vi "dfd_Draw Polynomial Matrix Element.vi"(4 "format control":T1={"variable"="z", "rendering options"={"coefficients ascending order"=FALSE, "render ascending order"=TRUE, "negative exponent"=TRUE}}, 5 "fonts input":T5(array[cluster]), 6 "alignment(left, top)":T4, 7 "format string":string="%#.4g", 9 "origin":cluster{"x":i16, "y":i16}, 10 "coefficients":dbl[](array[numeric])=[1.0, 2.0, 1.0, 0.0, 2.0] format="%.2f", 11 "picture in":picture) -> (1 "location":T3, 3 "picture out":picture)   [LabVIEW 2017, in "NI_DigFilter_Process.lvlib"]
uses:
  <vilib>/addons/Digital Filter Design/NI_DigFilter_Process.lvlib
  <vilib>/Analysis/polynomials.llb/Remove Zero Coefficients (DBL).vi
  <vilib>/Analysis/NI_AALPro.lvlib
panel:
  in  "desired font(user-specified font)":T2(ring)
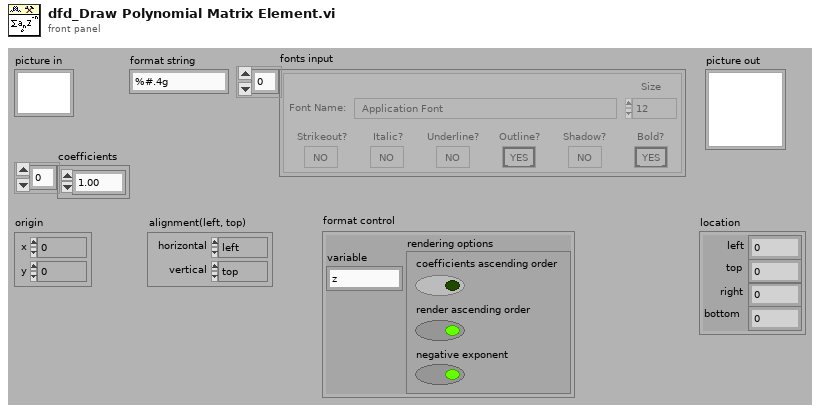
[diagram p1: front panel]
types:
  T1 = cluster{"variable":string, "rendering options":cluster{"coefficients ascending order":bool, "render ascending order":bool, "negative exponent":bool}}
  T2 = enum16{"User-specified Font", "Application Font", "System Font", "Dialog Font"}
  T3 = cluster{"left":i16, "top":i16, "right":i16, "bottom":i16}
  T4 = cluster{"horizontal":enum16{"left", "center", "right"}, "vertical":enum16{"top", "center", "bottom"}}
  T5 = cluster{"Font Name:":string, "Size":i16, "Strikeout?":bool, "Italic?":bool, "Underline?":bool, "Outline?":bool, "Shadow?":bool, "Bold?":bool}[]
  T6 = cluster{"Font Name:":string, "Size":i16, "Strikeout?":bool, "Italic?":bool, "Underline?":bool, "Outline?":bool, "Shadow?":bool, "Bold?":bool}
  T7 = cluster{"coefficients ascending order":bool, "render ascending order":bool, "negative exponent":bool}
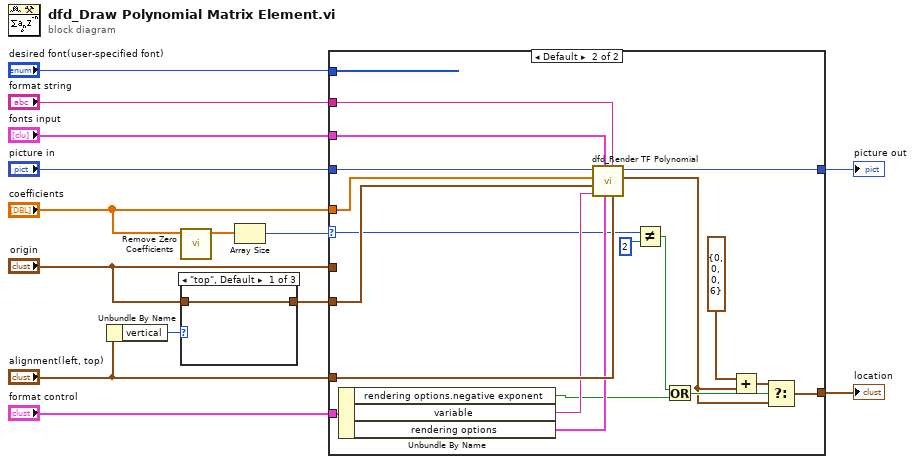
[diagram p0: block diagram]
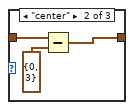
[diagram p2: hidden frame]
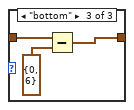
[diagram p3: hidden frame]
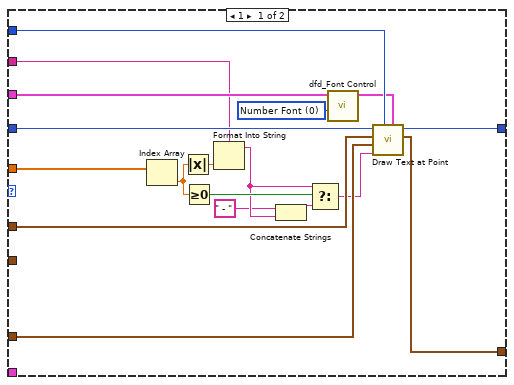
[diagram p4: hidden frame]
diagram:
  n1 = Unbundle By Name("alignment(left, top)") -> ("vertical"=w7:enum16{"top", "center", "bottom"})
  n2 = call-poly <vilib>:"Remove Zero Coefficients.vi"("P(x) In"="coefficients") -> ("P(x) Out"=w2:dbl[])  [unwired: 2 in, 8 out]
  n3 = case shown="\"top\", Default" w7 {
    tunnel: "origin" -> [w15 w17 w20]
    tunnel: [w15 w16 w19] -> w6
    frame "top", Default {
    }
    frame "center" {
      n4 = Subtract(x=w17, y=cluster{"x":i16, "y":i16} {"x"=0, "y"=3}) -> (x-y=w16:cluster{"x":i16, "y":i16})
    }
    frame "bottom" {
      n5 = Subtract(x=w20, y=cluster{"x":i16, "y":i16} {"x"=0, "y"=6}) -> (x-y=w19:cluster{"x":i16, "y":i16})
    }
  }
  n6 = Array Size(array=w2) -> (size(s)=w1:i32)
  n7 = case shown="Default" w1 {
    selector: w1 -> [_ w48]
    tunnel: "fonts input" -> [w33 w58]
    tunnel: "format string" -> [w29 w57]
    tunnel: "picture in" -> [w39 w56]
    tunnel: [w38 w55] -> w11
    tunnel: "alignment(left, top)" -> [w36 w54]
    tunnel: [w37 w43] -> w10
    tunnel: "coefficients" -> [w30 w53]
    tunnel: "desired font(user-specified font)" -> [w35 _]
    tunnel: w6 -> [_ w52]
    tunnel: "origin" -> [w31 _]
    tunnel: "format control" -> [_ w51]
    frame 1 {
      w34 = u16 0 items=["Number Font", "Variable Font", "Script Font"] ("Tpye")
      n8 = Index Array(array=w30) -> (element=w27:dbl)  [unwired: 1 in]
      n9 = Absolute Value(x=w27) -> (abs(x)=w28:dbl)
      n10 = Greater Or Equal To 0?(x=w27) -> (x >= 0?=w26:bool)
      n11 = Format Into String(format string=w29, w28) -> (resulting string=w24:string)  [unwired: 2 in, 1 out]
      n12 = Concatenate Strings(" - " ("string"), w24) -> (w23:string)
      n13 = Select(t=w24, s=w26, f=w23) -> (s? t:f=w25:string)
      n14 = call <vilib>:"dfd_Font Control.vi"("tpye"=w34, "fonts input"=w33) -> ("font output"=w32:T6)  [unwired: 9 out]
      n15 = call <vilib>:"Draw Text at Point.vi"("[user-specified font]"=w32, "desired font(Application)"=w35, "text"=w25, "alignment(left, top)"=w36, "origin"=w31, "picture"=w39) -> ("text rect"=w37:T3, "new picture"=w38:picture)  [unwired: 3 in, 1 out]
    }
    frame Default {
      n16 = Unbundle By Name(w51) -> ("rendering options.negative exponent"=w45:bool, "variable"=w50:string, "rendering options"=w49:T7)
      n17 = call <vilib>:"dfd_Render TF Polynomial.vi"("alignment(left, top)"=w54, "format string"=w57, "rendering options"=w49, "Fonts Input"=w58, "variable"=w50, "origin"=w52, "coefficients"=w53, "picture in"=w56) -> ("text rect"=w41:T3, "rendered equation"=w55:picture)  [unwired: 2 out]
      n18 = Not Equal?(x=w48, y=2) -> (x != y?=w46:bool)
      n19 = Or(x=w46, y=w45) -> (x .or. y?=w44:bool)
      n20 = Add(x=T3 {"left"=0, "top"=0, "right"=0, "bottom"=6} ("text rect"), y=w41) -> (x+y=w42:T3)
      n21 = Select(t=w42, s=w44, f=w41) -> (s? t:f=w43:T3)
    }
  }
  "picture out" <- w11
  "location" <- w10
